vi "GetDefectId.vi"(8 "error in":errorcluster, 11 "Defect in":refnum<class "Defect.lvclass">) -> (0 "error out":errorcluster, 2 "DefectId":string, 3 "Defect out":refnum<class "Defect.lvclass">)   [LabVIEW 2021, in "ProligentXMLGenerator.lvlib" / "Defect.lvclass"]
doc: "The ID of the current defect.\nThis attribute cannot be updated once sent to the DIT."
uses:
  Defect.lvclass
  Defect.lvclass/Defect.ctl
  Base/Guid/Guid.lvclass
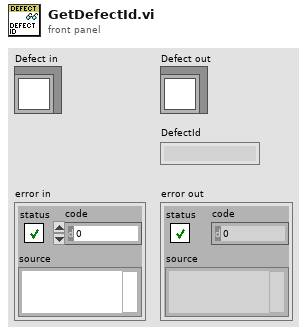
[diagram p1: front panel]
types:
  T1 = typedef "ProligentXMLGenerator.lvlib/Defect.lvclass/Data.ctl" = cluster{"Name":string, "Comments":refnum<class "UserComment.lvclass">[], "CustomData":refnum<class "CustomData.lvclass">, "DefectId":refnum<class "Guid.lvclass">, "OpenTime":refnum<class "DateTime.lvclass">, "TimeZoneInfoId":string}
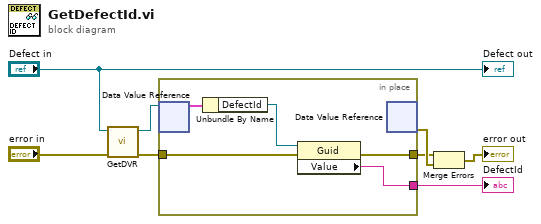
[diagram p0: block diagram]
diagram:
  n1 = call "GetDVR.vi"("error in"="error in", "Defect"="Defect in") -> ("error out"=w4:errorcluster, "DVRReference"=w7:refnum<data-value>)  [unwired: 8 in]
  n2 = in-place "In Place Element Structure" {
    in-place-border: w4 -> [w11]
    in-place-border: [w10] -> w3
    in-place-border: [w9] -> w1
    n3 = in-place-dvr #1(w7) -> (w13:T1)  [unwired: 1 out]
    n4 = Unbundle By Name(w13) -> ("DefectId"=w12:refnum<class "Guid.lvclass">)
    n5 = property on="Property Node" class="Guid"(reference=w12, error in=w11) -> (error out=w10:errorcluster, "Value"=w9:string)  [unwired: 1 out]
    n6 = in-place-dvr #1() -> (w8:errorcluster)  [unwired: 1 in, 1 out]
  }
  "DefectId" <- w1
  n7 = Merge Errors(w3, w8) -> (→"error out":errorcluster)
  "Defect out" <- "Defect in"
